vi "ztscopeM Init.vi"(0 "Resource Name":string, 1 "ID Query":i32(ring)=1 items=["Do Query"=1, "Skip Query"=0], 2 "Reset":i32(ring) items=["Reset Device"=1, "Don't Reset"=0], 3 "error in":errorcluster, 4 "Comm Bus":u16(ring)=2 items=["ZT_MCLASS"=2, "ZT_LAN"=4, "ZT_VISA_PCI_M"=258, "ZT_VISA_M"=514]) -> (7 "Instrument Handle":i32, 8 "Model Number":u32, 10 "error out":errorcluster)   [LabVIEW 2013]
doc: "Establish an instrument communication session."
uses:
  ztscopeM.dll
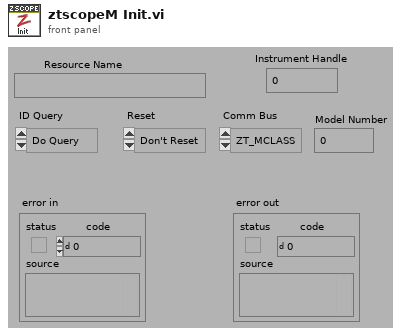
[diagram p1: front panel]
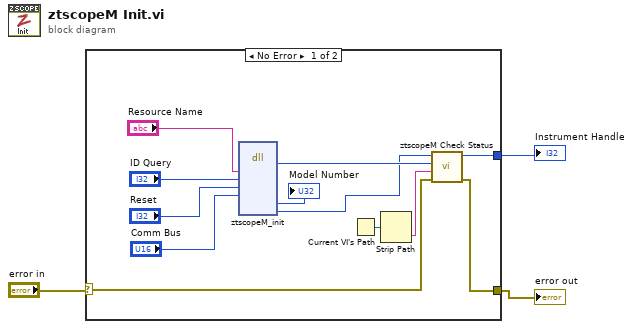
[diagram p0: block diagram]
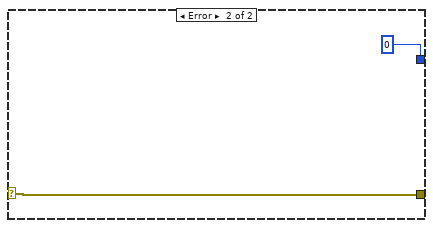
[diagram p2: hidden frame]
diagram:
  n1 = case shown="No Error" "error in" {
    selector: "error in" -> [w9 w16]
    tunnel: [w7 w16] -> w2
    tunnel: [w8 0 ("instrumentHandle")] -> w1
    frame No Error {
      n2 = dll-call lib="C:/Program Files/National Instruments/instr.lib/ztscopem/ztscopeM.dll" fn="ztscopeM_init"("resourceName"="Resource Name", "IDQuery"="ID Query", "reset"="Reset", "comm_bus"="Comm Bus") -> (w12:i32, "model_number"=→"Model Number":u32, "instrumentHandle"=w6:i32)  [unwired: 9 in, 2 out]
      n3 = Current VI's Path() -> (path=w11:path)
      n4 = Strip Path(path=w11) -> (name=w10:string)  [unwired: 1 out]
      n5 = call "ztscopeM Check Status.vi"("error in"=w9, "name of VI"=w10, "status"=w12, "instrument handle in"=w6) -> ("error out"=w7:errorcluster, "instrument handle out"=w8:i32)  [unwired: 2 in]
    }
    frame Error {
    }
  }
  "Instrument Handle" <- w1
  "error out" <- w2
